vi "Write keeper_plays.vi"(8 "error in (no error)":errorcluster, 10 "keeper_plays":T1, 11 "Playbook in":refnum<class "Playbook.lvclass">) -> (0 "error out":errorcluster, 3 "Playbook out":refnum<class "Playbook.lvclass">)   [LabVIEW 2023, in "Playbook.lvclass"]
uses:
  Playbook.lvclass
  keeper_plays.ctl
  Play_class/Play.lvclass
  TestPlay_class/TestPlay.lvclass
  HaltPlay_class/HaltPlay.lvclass
  KeeperPlay_class/KeeperPlay.lvclass
  TimeoutPlay_class/TimeoutPlay.lvclass
  ZigZagPlay_class/ZigZagPlay.lvclass
  GoToPlay_class/GoToPlay.lvclass
  Playbook.lvclass/Playbook.ctl
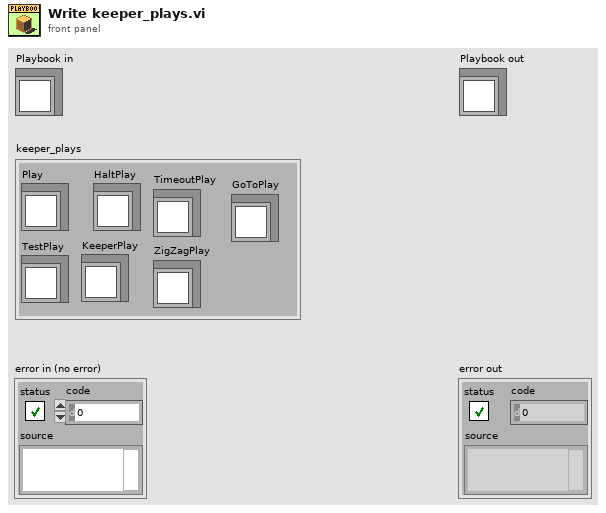
[diagram p1: front panel]
types:
  T1 = typedef "keeper_plays.ctl" = cluster{"Play":refnum<class "Play.lvclass">, "TestPlay":refnum<class "TestPlay.lvclass">, "HaltPlay":refnum<class "HaltPlay.lvclass">, "KeeperPlay":refnum<class "KeeperPlay.lvclass">, "TimeoutPlay":refnum<class "TimeoutPlay.lvclass">, "ZigZagPlay":refnum<class "ZigZagPlay.lvclass">, "GoToPlay":refnum<class "GoToPlay.lvclass">}
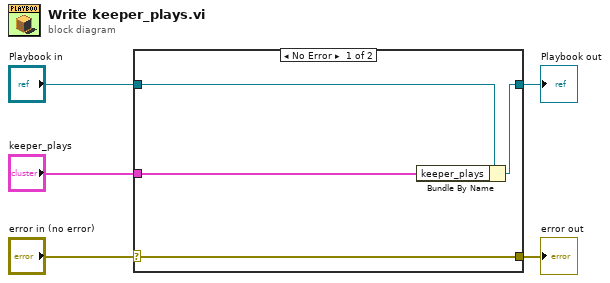
[diagram p0: block diagram]
diagram:
  n1 = case shown="No Error" "error in (no error)" {
    selector: "error in (no error)" -> [w9 w10]
    tunnel: [w9 w10] -> w4
    tunnel: [w7 w11] -> w2
    tunnel: "Playbook in" -> [w8 w11]
    tunnel: "keeper_plays" -> [w6 _]
    frame No Error {
      n2 = Bundle By Name(cluster=w8, "keeper_plays"=w6) -> (w7:refnum<class "Playbook.lvclass">)
    }
    frame Error {
    }
  }
  "error out" <- w4
  "Playbook out" <- w2
